vi "SQLite Error.vi"(6 "ID string":string, 8 "return type":i32, 9 "error in (no error)":errorcluster) -> (0 "error out":errorcluster)   [LabVIEW 2013, in "SQLiteSupport.lvlib"]
uses:
  SQLiteSupport.lvlib
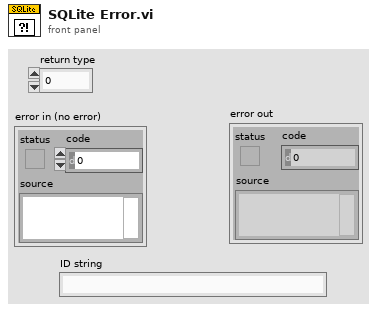
[diagram p1: front panel]
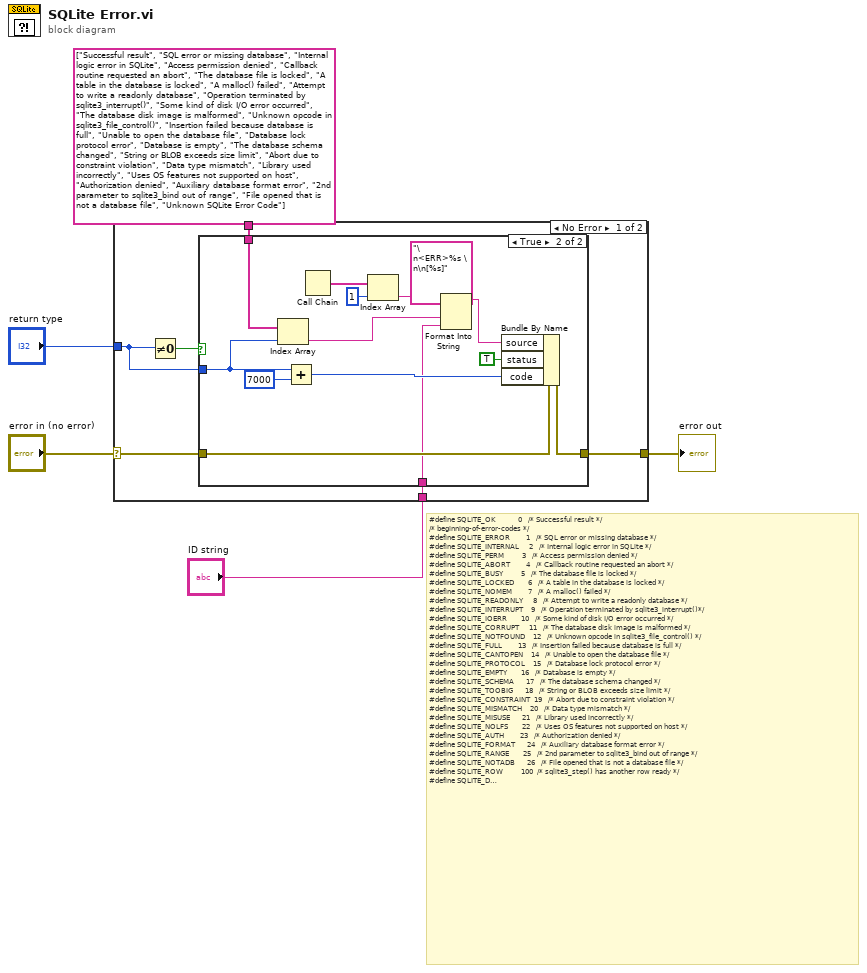
[diagram p0: block diagram]
diagram:
  # "#define SQLITE_OK           0   /* Successful result */\n/* beginning-of-error-codes */\n#define SQLITE_ERROR        1   /* SQL error or missing database */\n#define SQLITE_INTERNAL     2   /* Internal logic error in SQLite */\n#define SQLITE_PERM         3   /* Access permission denied */\n#define SQLITE_ABORT        4   /* Callback routine requested an abort */\n#define SQLITE_BUSY         5   /* The database file is locked */\n#define SQLITE_LOCKED       6   /* A table in the database is locked */\n#define SQLITE_NOMEM        7   /* A malloc() failed */\n#define SQLITE_READONLY     8   /* Attempt to write a readonly database */\n#define SQLITE_INTERRUPT    9   /* Operation terminated by sqlite3_interrupt()*/\n#define SQLITE_IOERR       10   /* Some kind of disk I/O error occurred */\n#define SQLITE_CORRUPT     11   /* The database disk image is malformed */\n#define SQLITE_NOTFOUND    12   /* Unknown opcode in sqlite3_file_control() */\n#define SQLITE_FULL        13   /* Insertion failed because database is full */\n#define SQLITE_CANTOPEN    14   /* Unable to open the database file */\n#define SQLITE_PROTOCOL    15   /* Database lock protocol error */\n#define SQLITE_EMPTY       16   /* Database is empty */\n#define SQLITE_SCHEMA      17   /* The database schema changed */\n#define SQLITE_TOOBIG      18   /* String or BLOB exceeds size limit */\n#define SQLITE_CONSTRAINT  19   /* Abort due to constraint violation */\n#define SQLITE_MISMATCH    20   /* Data type mismatch */\n#define SQLITE_MISUSE      21   /* Library used incorrectly */\n#define SQLITE_NOLFS       22   /* Uses OS features not supported on host */\n#define SQLITE_AUTH        23   /* Authorization denied */\n#define SQLITE_FORMAT      24   /* Auxiliary database format error */\n#define SQLITE_RANGE       25   /* 2nd parameter to sqlite3_bind out of range */\n#define SQLITE_NOTADB      26   /* File opened that is not a database file */\n#define SQLITE_ROW         100  /* sqlite3_step() has another row ready */\n#define SQLITE_DONE        101  /* sqlite3_step() has finished executing */"
  n1 = case shown="No Error" "error in (no error)" {
    selector: "error in (no error)" -> [w9 w27]
    tunnel: "return type" -> [w10 _]
    tunnel: [w8 w27] -> w4
    tunnel: string[] ["Successful result", "SQL error or missing database", "Internal logic error in SQLite", "Access permission denied", "Callback routine requested an abort", "The database file is locked", "A table in the database is locked", "A malloc() failed", "Attempt to write a readonly database", "Operation terminated by sqlite3_interrupt()", "Some kind of disk I/O error occurred", "The database disk image is malformed", "Unknown opcode in sqlite3_file_control()", "Insertion failed because database is full", "Unable to open the database file", "Database lock protocol error", "Database is empty", "The database schema changed", "String or BLOB exceeds size limit", "Abort due to constraint violation", "Data type mismatch", "Library used incorrectly", "Uses OS features not supported on host", "Authorization denied", "Auxiliary database format error", "2nd parameter to sqlite3_bind out of range", "File opened that is not a database file", "Unknown SQLite Error Code"] ("Array") -> [w7 _]
    tunnel: "ID string" -> [w6 _]
    frame No Error {
      n2 = Not Equal To 0?(x=w10) -> (x != 0?=w11:bool)
      n3 = case shown="True" w11 {
        tunnel: w10 -> [_ w20]
        tunnel: w9 -> [w12 w26]
        tunnel: [w12 w25] -> w8
        tunnel: w7 -> [_ w21]
        tunnel: w6 -> [_ w13]
        frame False {
        }
        frame True {
          n4 = Index Array(array=w21, index=w20) -> (element=w16:string)
          n5 = Add(x=w20, y=7000) -> (x+y=w24:i32)
          n6 = Call Chain() -> (call chain=w18:string[])
          n7 = Index Array(array=w18, index=1) -> (element=w17:string)
          n8 = Format Into String(format string="\n<ERR>%s \n\n[%s]", initial string=w17, w16, w13) -> (resulting string=w14:string)  [unwired: 1 in, 1 out]
          n9 = Bundle By Name(cluster=w26, "source"=w14, "status"=TRUE, "code"=w24) -> (w25:errorcluster)
        }
      }
    }
    frame Error {
    }
  }
  "error out" <- w4
